vi "Apply Settings.vi"(8 "error in (no error)":errorcluster, 11 "Electronic Load in":refnum<class "Electronic Load.lvclass">) -> (0 "error out":errorcluster, 3 "Electronic Load out":refnum<class "Electronic Load.lvclass">)   [LabVIEW 2019, in "Electronic Load.lvlib" / "Electronic Load.lvclass"]
uses:
  Library/Electronic Load.lvclass
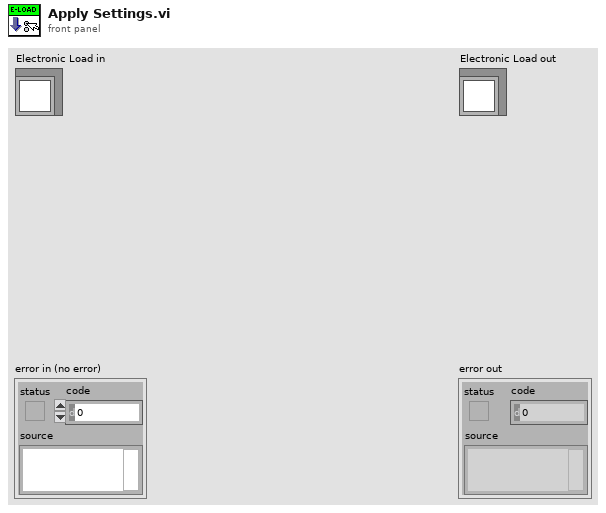
[diagram p1: front panel]
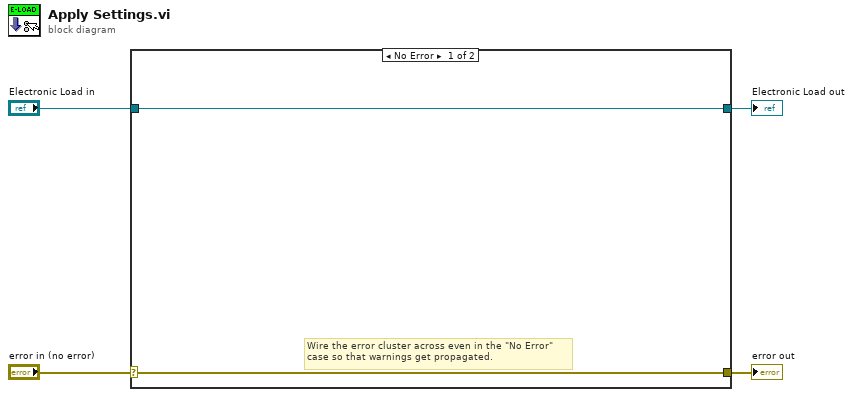
[diagram p0: block diagram]
diagram:
  n1 = case shown="No Error" "error in (no error)" {
    selector: "error in (no error)" -> [w5 w8]
    tunnel: [w5 w8] -> w3
    tunnel: [w6 w7] -> w1
    tunnel: "Electronic Load in" -> [w6 w7]
    frame No Error {
      # "Wire the error cluster across even in the \"No Error\"\ncase so that warnings get propagated."
    }
    frame Error {
    }
  }
  "error out" <- w3
  "Electronic Load out" <- w1
